vi "Obtain Doc Win ID.vi"(8 "error in (no error)":errorcluster, 11 "Py Doc in":refnum<class "Py Doc.lvclass">) -> (0 "error out":errorcluster, 3 "Py Doc out":refnum<class "Py Doc.lvclass">)   [LabVIEW 2019, in "Py Doc.lvclass"]
doc: "Set the specified window state.(Window Hide-0,Window Display -5)"
uses:
  Py Doc.lvclass
  D:/Namratha/MDI/LabVIEW-MDI-develop_LV2019/source code/Document/Document base/Document.lvclass
  Document base/Document.lvclass/Document.ctl
  Document base/property/Read Doc Title.vi
  Document base/property/Write Doc Hwnd.vi
  Document base/Document.lvclass
  MDI Library/LV MDI.lvclass
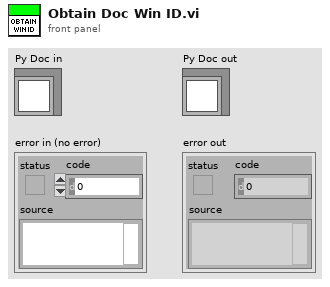
[diagram p1: front panel]
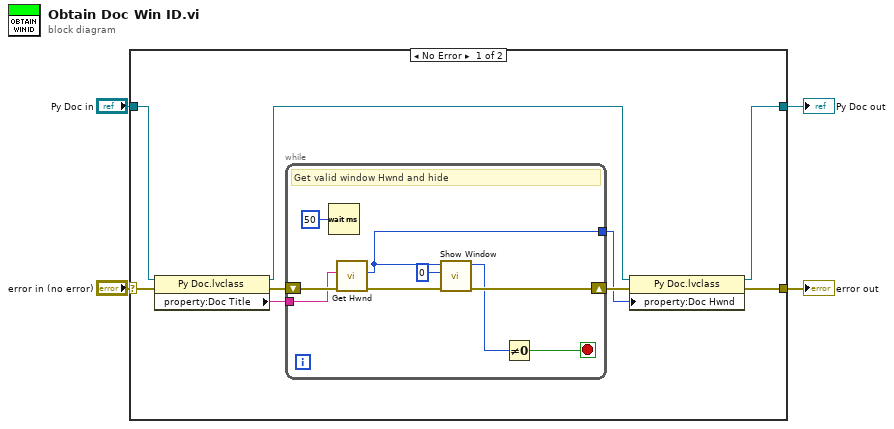
[diagram p0: block diagram]
diagram:
  n1 = case shown="No Error" "error in (no error)" {
    selector: "error in (no error)" -> [w12 w23]
    tunnel: [w8 w23] -> w3
    tunnel: "Py Doc in" -> [w10 w24]
    tunnel: [w6 w24] -> w1
    frame No Error {
      n2 = property class="Py Doc.lvclass"(reference=w10, error in=w12) -> (reference out=w7:refnum<class "Py Doc.lvclass">, error out=w11:errorcluster, "property:Doc Title"=w9:string)
      n3 = while {
        tunnel: w9 -> [w14]
        shift-right: [w19] -> w13
        shift-left: w11 -> [w15]
        tunnel: [w17] -> w5
        stop <- w21 stop-if-true
        # "Get valid window Hwnd and hide"
        n4 = Wait (ms)(milliseconds to wait=u32 50) -> ()  [unwired: 1 out]
        n5 = call "Get Hwnd.vi"("error in (no error)"=w15, "Doc Name"=w14) -> ("error out"=w16:errorcluster, "hwnd"=w17:u32)  [unwired: 8 in]
        n6 = call "Show Window.vi"("error in (no error)"=w16, "Window State"=u32 0 ("nCmdShow"), "hwnd"=w17) -> ("error out"=w19:errorcluster, "Wnd previously Visible?"=w18:u32)  [unwired: 7 in]
        n7 = Not Equal To 0?(x=w18) -> (x != 0?=w21:bool)
      }
      n8 = property class="Py Doc.lvclass"(reference=w7, error in=w13, "property:Doc Hwnd"=w5) -> (reference out=w6:refnum<class "Py Doc.lvclass">, error out=w8:errorcluster)
    }
    frame Error {
    }
  }
  "error out" <- w3
  "Py Doc out" <- w1
